vi "设置自动快门间隔.vi"(8 "error in":errorcluster, 10 "时间间隔设置":T1={"快门第一次延时时间"=200, "快门第二次延时时间"=200, "切换增益后快门第一次延时时间"=200, "切换增益后快门第二次延时时间"=200}) -> (0 "error out":errorcluster, 2 "return":i32)   [LabVIEW 2016]
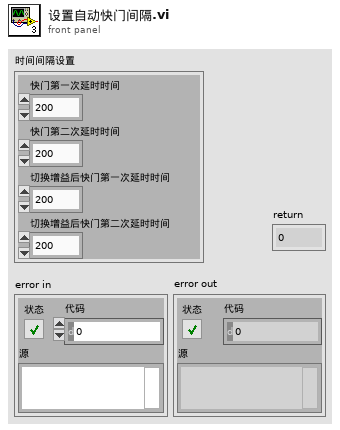
[diagram p1: front panel]
types:
  T1 = cluster{"快门第一次延时时间":u16, "快门第二次延时时间":u16, "切换增益后快门第一次延时时间":u16, "切换增益后快门第二次延时时间":u16}
  T2 = cluster{"byCmdType":u8, "bySubCmd":u8, "byParam_h":u8, "byParam_l":u8, "byAddr1_hh":u8, "byAddr1_h":u8, "byAddr1_l":u8, "byAddr1_ll":u8, "byAddr2_hh":u8, "byAddr2_h":u8, "byAddr2_l":u8, "byAddr2_ll":u8, "byLen_hh":u8, "byLen_h":u8, "byLen_l":u8, "byLen_ll":u8}
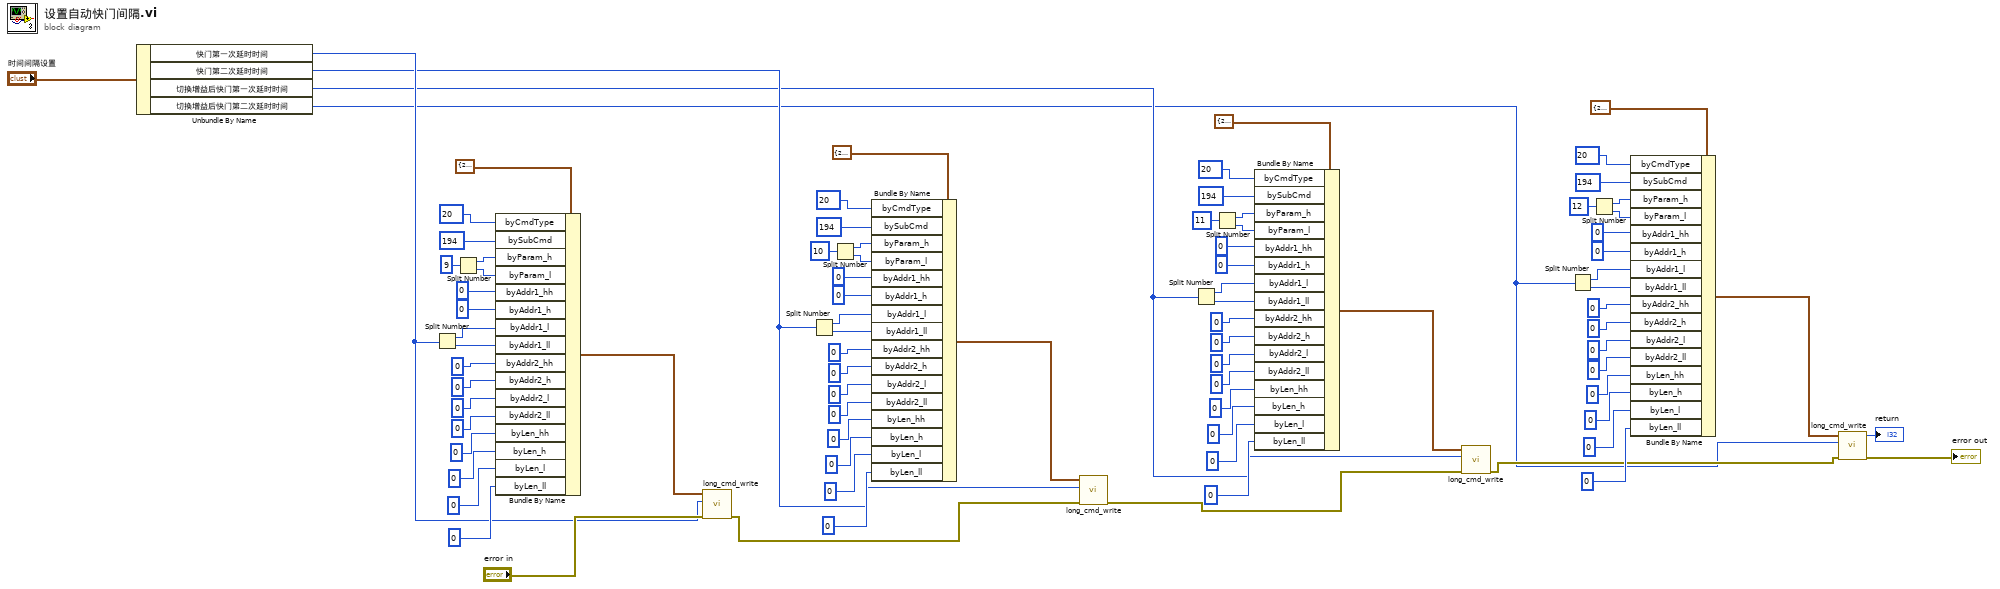
[diagram p0: block diagram]
diagram:
  n1 = Unbundle By Name("时间间隔设置") -> ("快门第一次延时时间"=w4:u16, "快门第二次延时时间"=w3:u16, "切换增益后快门第一次延时时间"=w2:u16, "切换增益后快门第二次延时时间"=w1:u16)
  n2 = Split Number(x=w4) -> (hi(x)=w78:u8, lo(x)=w77:u8)
  n3 = Split Number(x=u8 9 ("byParam_h")) -> (hi(x)=w83:u8, lo(x)=w81:u8)
  n4 = Bundle By Name(cluster=T2 {"byCmdType"=24, "bySubCmd"=129, "byParam_h"=0, "byParam_l"=0, "byAddr1_hh"=0, "byAddr1_h"=0, "byAddr1_l"=0, "byAddr1_ll"=0, "byAddr2_hh"=0, "byAddr2_h"=0, "byAddr2_l"=0, "byAddr2_ll"=0, "byLen_hh"=0, "byLen_h"=0, "byLen_l"=0, "byLen_ll"=0} ("vd_cmd_long_header_t"), "byCmdType"=20, "bySubCmd"=194, "byParam_h"=w83, "byParam_l"=w81, "byAddr1_hh"=u8 0 ("byParam_h"), "byAddr1_h"=u8 0 ("byParam_h"), "byAddr1_l"=w78, "byAddr1_ll"=w77, "byAddr2_hh"=u8 0 ("byParam_h"), "byAddr2_h"=u8 0 ("byParam_h"), "byAddr2_l"=u8 0 ("byParam_h"), "byAddr2_ll"=u8 0 ("byParam_h"), "byLen_hh"=u8 0 ("byParam_h"), "byLen_h"=u8 0 ("byParam_h"), "byLen_l"=u8 0 ("byParam_h"), "byLen_ll"=u8 0 ("byParam_h")) -> (w84:T2)
  n5 = call "long_cmd_write.vi"("error in"="error in", "dwAddr1"=w4, "vd_cmd_long_header_t"=w84) -> ("error out"=w11:errorcluster)  [unwired: 7 in, 1 out]
  n6 = Split Number(x=w3) -> (hi(x)=w59:u8, lo(x)=w60:u8)
  n7 = Split Number(x=u8 10 ("byParam_h")) -> (hi(x)=w54:u8, lo(x)=w56:u8)
  n8 = Bundle By Name(cluster=T2 {"byCmdType"=24, "bySubCmd"=129, "byParam_h"=0, "byParam_l"=0, "byAddr1_hh"=0, "byAddr1_h"=0, "byAddr1_l"=0, "byAddr1_ll"=0, "byAddr2_hh"=0, "byAddr2_h"=0, "byAddr2_l"=0, "byAddr2_ll"=0, "byLen_hh"=0, "byLen_h"=0, "byLen_l"=0, "byLen_ll"=0} ("vd_cmd_long_header_t"), "byCmdType"=20, "bySubCmd"=194, "byParam_h"=w54, "byParam_l"=w56, "byAddr1_hh"=u8 0 ("byParam_h"), "byAddr1_h"=u8 0 ("byParam_h"), "byAddr1_l"=w59, "byAddr1_ll"=w60, "byAddr2_hh"=u8 0 ("byParam_h"), "byAddr2_h"=u8 0 ("byParam_h"), "byAddr2_l"=u8 0 ("byParam_h"), "byAddr2_ll"=u8 0 ("byParam_h"), "byLen_hh"=u8 0 ("byParam_h"), "byLen_h"=u8 0 ("byParam_h"), "byLen_l"=u8 0 ("byParam_h"), "byLen_ll"=u8 0 ("byParam_h")) -> (w53:T2)
  n9 = call "long_cmd_write.vi"("error in"=w11, "dwAddr1"=w3, "vd_cmd_long_header_t"=w53) -> ("error out"=w10:errorcluster)  [unwired: 7 in, 1 out]
  n10 = Split Number(x=w2) -> (hi(x)=w21:u8, lo(x)=w22:u8)
  n11 = Split Number(x=u8 11 ("byParam_h")) -> (hi(x)=w16:u8, lo(x)=w18:u8)
  n12 = Bundle By Name(cluster=T2 {"byCmdType"=24, "bySubCmd"=129, "byParam_h"=0, "byParam_l"=0, "byAddr1_hh"=0, "byAddr1_h"=0, "byAddr1_l"=0, "byAddr1_ll"=0, "byAddr2_hh"=0, "byAddr2_h"=0, "byAddr2_l"=0, "byAddr2_ll"=0, "byLen_hh"=0, "byLen_h"=0, "byLen_l"=0, "byLen_ll"=0} ("vd_cmd_long_header_t"), "byCmdType"=20, "bySubCmd"=194, "byParam_h"=w16, "byParam_l"=w18, "byAddr1_hh"=u8 0 ("byParam_h"), "byAddr1_h"=u8 0 ("byParam_h"), "byAddr1_l"=w21, "byAddr1_ll"=w22, "byAddr2_hh"=u8 0 ("byParam_h"), "byAddr2_h"=u8 0 ("byParam_h"), "byAddr2_l"=u8 0 ("byParam_h"), "byAddr2_ll"=u8 0 ("byParam_h"), "byLen_hh"=u8 0 ("byParam_h"), "byLen_h"=u8 0 ("byParam_h"), "byLen_l"=u8 0 ("byParam_h"), "byLen_ll"=u8 0 ("byParam_h")) -> (w15:T2)
  n13 = call "long_cmd_write.vi"("error in"=w10, "dwAddr1"=w2, "vd_cmd_long_header_t"=w15) -> ("error out"=w9:errorcluster)  [unwired: 7 in, 1 out]
  n14 = Split Number(x=w1) -> (hi(x)=w40:u8, lo(x)=w39:u8)
  n15 = Split Number(x=u8 12 ("byParam_h")) -> (hi(x)=w45:u8, lo(x)=w43:u8)
  n16 = Bundle By Name(cluster=T2 {"byCmdType"=24, "bySubCmd"=129, "byParam_h"=0, "byParam_l"=0, "byAddr1_hh"=0, "byAddr1_h"=0, "byAddr1_l"=0, "byAddr1_ll"=0, "byAddr2_hh"=0, "byAddr2_h"=0, "byAddr2_l"=0, "byAddr2_ll"=0, "byLen_hh"=0, "byLen_h"=0, "byLen_l"=0, "byLen_ll"=0} ("vd_cmd_long_header_t"), "byCmdType"=20, "bySubCmd"=194, "byParam_h"=w45, "byParam_l"=w43, "byAddr1_hh"=u8 0 ("byParam_h"), "byAddr1_h"=u8 0 ("byParam_h"), "byAddr1_l"=w40, "byAddr1_ll"=w39, "byAddr2_hh"=u8 0 ("byParam_h"), "byAddr2_h"=u8 0 ("byParam_h"), "byAddr2_l"=u8 0 ("byParam_h"), "byAddr2_ll"=u8 0 ("byParam_h"), "byLen_hh"=u8 0 ("byParam_h"), "byLen_h"=u8 0 ("byParam_h"), "byLen_l"=u8 0 ("byParam_h"), "byLen_ll"=u8 0 ("byParam_h")) -> (w46:T2)
  n17 = call "long_cmd_write.vi"("error in"=w9, "dwAddr1"=w1, "vd_cmd_long_header_t"=w46) -> ("error out"=→"error out":errorcluster, "return"=→"return":i32)  [unwired: 7 in]
